vi "Initialize.vi"(8 "error in":errorcluster, 11 "Plugin in":refnum<class "StreamReader.lvclass">) -> (0 "error out":errorcluster, 3 "Plugin out":refnum<class "StreamReader.lvclass">)   [LabVIEW 2024, in "StreamReader.lvlib" / "StreamReader.lvclass"]
uses:
  StreamReader.lvclass
  C:/Program Files/National Instruments/LabVIEW 2024/vi.lib/FlexLogger/SDK/PluginSDK.lvlibp/PEFClasses/SDK/Plugin/Plugin.lvclass
  StreamReader Strings.vi
  <vilib>/FlexLogger/SDK/PluginSDK.lvlibp/PEFClasses/SDK/Plugin/ParameterAccess/Write String.vi
  <vilib>/FlexLogger/SDK/PluginSDK.lvlibp/PEFClasses/SDK/Plugin/ParameterAccess/Write I32.vi
  <vilib>/FlexLogger/SDK/PluginSDK.lvlibp/PEFClasses/SDK/Plugin/Plugin.lvclass
  C:/Program Files/National Instruments/LabVIEW 2024/vi.lib/FlexLogger/SDK/PluginSDK.lvlibp/PEFClasses/SDK/Processing Element/Processing Element.lvclass
  C:/Users/Administrator/Documents/LabVIEW Projects/FlexLogger IO Plug-ins/StreamReader/StreamReader.lvclass
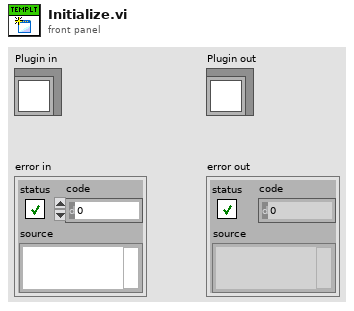
[diagram p1: front panel]
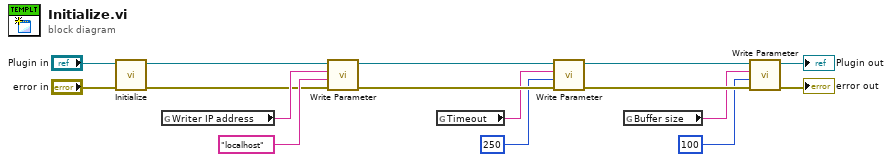
[diagram p0: block diagram]
diagram:
  n1 = call-parent "Initialize.vi"("error in (no error)"="error in", "Plugin in"="Plugin in") -> ("error out"=w1:errorcluster, "Plugin out"=w2:refnum<class "StreamReader.lvclass">)  [unwired: 8 in]
  n2 = global read "StreamReader Strings.vi" "Writer IP address"() -> (w7:string)
  n3 = call-poly <vilib>:"Write Parameter.vi"("error in (no error)"=w1, "Value"="localhost", "Name"=w7, "Plugin in"=w2) -> ("error out"=w13:errorcluster, "Plugin out"=w14:refnum<class "StreamReader.lvclass">)  [unwired: 6 in]
  n4 = global read "StreamReader Strings.vi" "Timeout"() -> (w5:string)
  n5 = call-poly <vilib>:"Write Parameter.vi"("error in (no error)"=w13, "Value"=250, "Name"=w5, "Plugin in"=w14) -> ("error out"=w11:errorcluster, "Plugin out"=w12:refnum<class "StreamReader.lvclass">)  [unwired: 6 in]
  n6 = global read "StreamReader Strings.vi" "Buffer size"() -> (w6:string)
  n7 = call-poly <vilib>:"Write Parameter.vi"("error in (no error)"=w11, "Value"=100, "Name"=w6, "Plugin in"=w12) -> ("error out"=→"error out":errorcluster, "Plugin out"=→"Plugin out":refnum<class "StreamReader.lvclass">)  [unwired: 6 in]
